vi "Get SelectedItem Index.vi"(8 "error in (no error)":errorcluster caption="错误输入（无错误）", 11 "ListViewClass 输入":refnum<class "ListViewClass.lvclass"> caption="DNL_LabVIEW Object in") -> (0 "error out":errorcluster caption="错误输出", 2 "Selected Index":i32[](array[numeric]), 3 "ListViewClass 输出":refnum<class "ListViewClass.lvclass"> caption="DNL_LabVIEW Object out")   [LabVIEW 2012, in "ListViewClass.lvclass"]
uses:
  ListViewClass.lvclass
  ListViewClass.lvclass/ListViewClass.ctl
  System.Windows.Forms
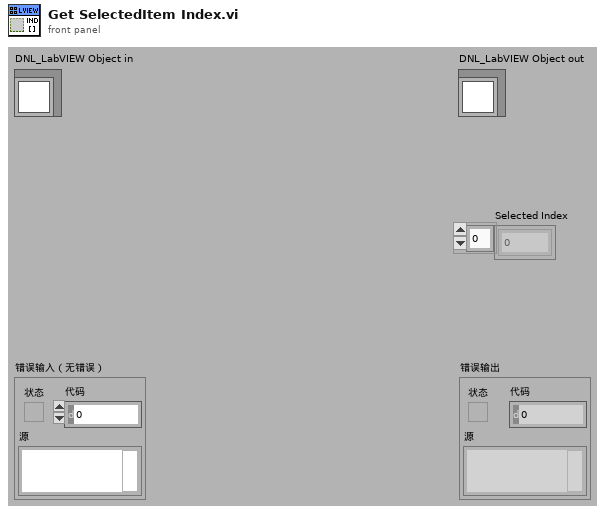
[diagram p1: front panel]
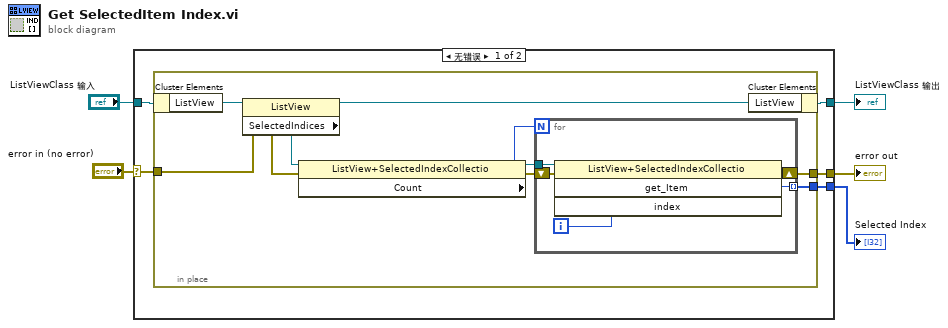
[diagram p0: block diagram]
diagram:
  n1 = case shown="无错误" "error in (no error)" {
    selector: "error in (no error)" -> [w9 w27]
    tunnel: [w8 w27] -> w4
    tunnel: [w7 w26] -> w2
    tunnel: "ListViewClass 输入" -> [w10 w26]
    tunnel: [w6 _] -> w1
    frame No Error {
      n2 = in-place {
        in-place-border: w9 -> [w15]
        in-place-border: [w12] -> w8
        in-place-border: [w11] -> w6
        n3 = in-place-cluster #1(w10) -> ("ListView"=w20:refnum<k24>)
        n4 = property class="ListView"(reference=w20, error in=w15) -> (reference out=w19:refnum<k24>, error out=w14:errorcluster, "SelectedIndices"=w18:refnum<k24>)
        n5 = property class="ListView+SelectedIndexCollectio"(reference=w18, error in=w14) -> (reference out=w17:refnum<k24>, error out=w13:errorcluster, "Count"=w16:i32)
        n6 = for {
          N: w16 -> [_]
          tunnel: w17 -> [w25]
          shift-right: [w22] -> w12
          shift-left: w13 -> [w23]
          tunnel: [w21] -> w11 mode=indexing
          i -> [w24]
          n7 = invoke class="ListView+SelectedIndexCollectio" method="get_Item"(reference=w25, error in=w23, "index"=w24) -> (error out=w22:errorcluster, "get_Item"=w21:i32)  [unwired: 1 in, 2 out]
        }
        n8 = in-place-cluster #1("ListView"=w19) -> (w7:refnum<class "ListViewClass.lvclass">)
      }
    }
    frame Error {
    }
  }
  "error out" <- w4
  "ListViewClass 输出" <- w2
  "Selected Index" <- w1
